vi "FPGA_AIReadOversampleBits.vi"(8 "error in (no error)":errorcluster, 9 "Additional Depth":i32, 10 "Channel":T1=enum."Invalid", 11 "AI Reference in":T2) -> (0 "error out":errorcluster, 2 "OversampleBits":u8, 3 "AI Reference out":T2)   [LabVIEW 2017]
uses:
  <vilib>/Rock Robotics/SystemInterfaces/AI/FPGA_AIDevRef.ctl
  <vilib>/Rock Robotics/SystemInterfaces/AI/FPGA_AIChannel.ctl
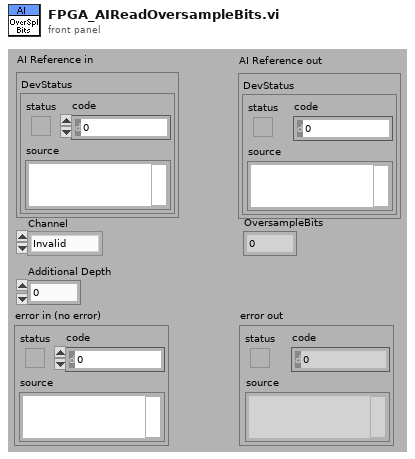
[diagram p1: front panel]
types:
  T1 = typedef "FPGA_AIChannel.ctl" = enum8{"AI 0", "AI 1", "AI 2", "AI 3", "AI MXP 0", "AI MXP 1", "AI MXP 2", "AI MXP 3", "Invalid"}
  T2 = typedef "FPGA_AIDevRef.ctl" = cluster{"DevStatus":errorcluster}
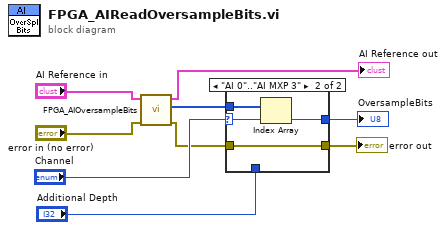
[diagram p0: block diagram]
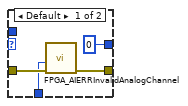
[diagram p2: hidden frame]
diagram:
  n1 = call <vilib>:"FPGA_AIOversampleBits.vi"("error in (no error)"="error in (no error)", "AI Reference in"="AI Reference in") -> ("error out"=w3:errorcluster, "OversampleBits out"=w7:u8[], "AI Reference out"=→"AI Reference out":T2)  [unwired: 2 in, 5 out]
  n2 = case shown="\"AI 0\"..\"AI MXP 3\"" "Channel" {
    selector: "Channel" -> [_ w16]
    tunnel: w7 -> [_ w17]
    tunnel: [u8 0 ("AverageBits") w15] -> w4
    tunnel: w3 -> [w12 w14]
    tunnel: [w11 w14] -> w2
    tunnel: "Additional Depth" -> [w10 _]
    frame Default {
      n3 = call <vilib>:"FPGA_AIERRInvalidAnalogChannel.vi"("error in (no error)"=w12, "Additional Depth"=w10) -> ("error out"=w11:errorcluster)  [unwired: 9 in]
    }
    frame "AI 0".."AI MXP 3" {
      n4 = Index Array(array=w17, index=w16) -> (element=w15:u8)
    }
  }
  "OversampleBits" <- w4
  "error out" <- w2
